vi "Update Flags.vi"(8 "error in (no error)":errorcluster, 10 "Flags":T1[](array[typedef]), 11 "Tosca in":refnum<class "Parameters.lvclass">) -> (0 "error out":errorcluster, 3 "Tosca out":refnum<class "Parameters.lvclass">)   [LabVIEW 2015, in "Parameters.lvclass"]
uses:
  Parameters.lvclass
  Typedefs/Tosca-Flag.ctl
  Parameters.lvclass/Parameters.ctl
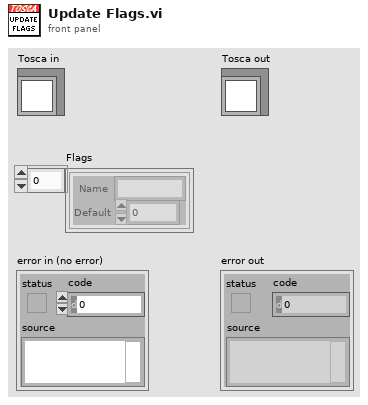
[diagram p1: front panel]
types:
  T1 = typedef "Tosca-Flag.ctl" = cluster{"Name":string, "Default":i32}
  T2 = typedef "Tosca-Input Event.ctl" = cluster{"Name":string, "Criteria":T3[], "Operators":enum16{"AND", "OR"}[], "Accumulator":T5}
  T3 = typedef "Tosca-Input Criterion.ctl" = cluster{"DigInput":i32, "State":T4, "Time (ms)":i32, "Name":string}
  T4 = typedef "Logic State.ctl" = enum16{"Low", "High", "Rising", "Falling"}
  T5 = typedef "Tosca-Accumulator.ctl" = cluster{"active":bool, "N":i32, "T":dbl, "Imax":dbl, "latency":dbl}
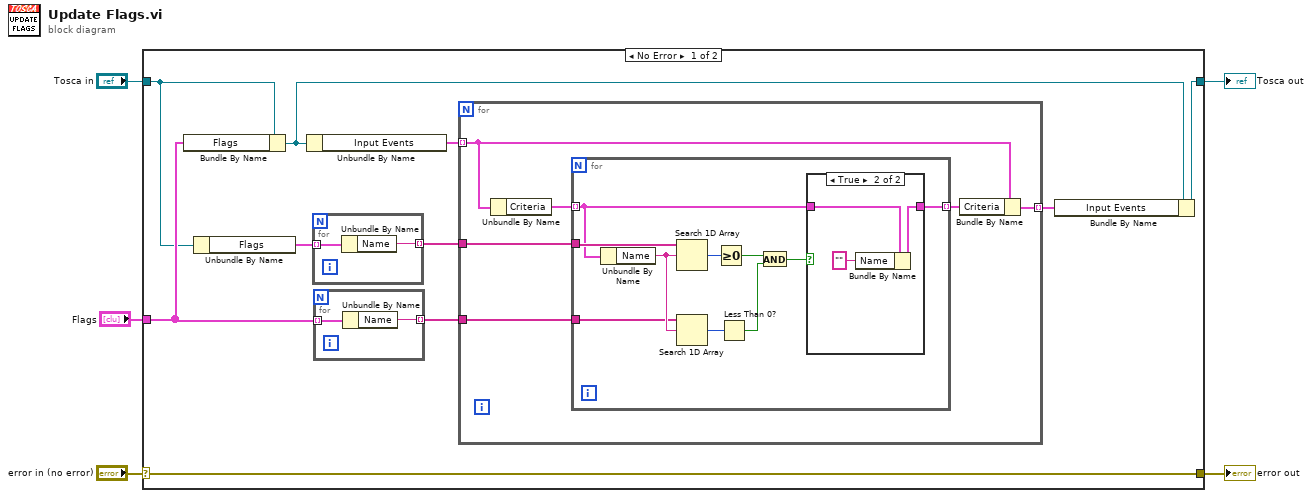
[diagram p0: block diagram]
diagram:
  n1 = case shown="No Error" "error in (no error)" {
    selector: "error in (no error)" -> [w15 w41]
    tunnel: [w15 w41] -> w4
    tunnel: [w8 w40] -> w2
    tunnel: "Tosca in" -> [w7 w40]
    tunnel: "Flags" -> [w11 _]
    frame No Error {
      n2 = Bundle By Name(cluster=w7, "Flags"=w11) -> (w6:refnum<class "Parameters.lvclass">)
      n3 = Unbundle By Name(w7) -> ("Flags"=w13:T1[])
      n4 = Unbundle By Name(w6) -> ("Input Events"=w14:T2[])
      n5 = for {
        tunnel: w13 -> [w19] mode=indexing
        tunnel: [w18] -> w12 mode=indexing
        n6 = Unbundle By Name(w19) -> ("Name"=w18:string)
      }
      n7 = for {
        tunnel: w11 -> [w17] mode=indexing
        tunnel: [w16] -> w10 mode=indexing
        n8 = Unbundle By Name(w17) -> ("Name"=w16:string)
      }
      n9 = for {
        tunnel: w14 -> [w22] mode=indexing
        tunnel: w12 -> [w24]
        tunnel: w10 -> [w23]
        tunnel: [w20] -> w9 mode=indexing
        n10 = Unbundle By Name(w22) -> ("Criteria"=w25:T3[])
        n11 = for {
          tunnel: w25 -> [w27] mode=indexing
          tunnel: w24 -> [w35]
          tunnel: w23 -> [w33]
          tunnel: [w26] -> w21 mode=indexing
          n12 = Unbundle By Name(w27) -> ("Name"=w34:string)
          n13 = Search 1D Array(1D array=w35, element=w34) -> (index of element=w32:i32)  [unwired: 1 in]
          n14 = Search 1D Array(1D array=w33, element=w34) -> (index of element=w31:i32)  [unwired: 1 in]
          n15 = Greater Or Equal To 0?(x=w32) -> (x >= 0?=w30:bool)
          n16 = Less Than 0?(x=w31) -> (x < 0?=w29:bool)
          n17 = And(x=w30, y=w29) -> (x .and. y?=w28:bool)
          n18 = case shown="True" w28 {
            tunnel: w27 -> [w36 w39]
            tunnel: [w36 w37] -> w26
            frame False {
            }
            frame True {
              n19 = Bundle By Name(cluster=w39, "Name"="") -> (w37:T3)
            }
          }
        }
        n20 = Bundle By Name(cluster=w22, "Criteria"=w21) -> (w20:T2)
      }
      n21 = Bundle By Name(cluster=w6, "Input Events"=w9) -> (w8:refnum<class "Parameters.lvclass">)
    }
    frame Error {
    }
  }
  "error out" <- w4
  "Tosca out" <- w2
